vi "Read Channel Configurations.vi"(8 "error in (no error)":errorcluster, 9 "PMU Configuration":T4, 10 "PMU Index":i32, 11 "Pseudo PDC ID":i32) -> (0 "error out":errorcluster, 1 "Digital Configuration":T1, 2 "Analog Configuration":T2, 3 "Phasor Configuration":T3)   [LabVIEW 2018, in "S3DK.lvlib" / "PMU Recorder Light.lvlib" / "Statnett C37.118 DLL.lvclass"]
uses:
  Statnett C37.118 DLL.lvclass
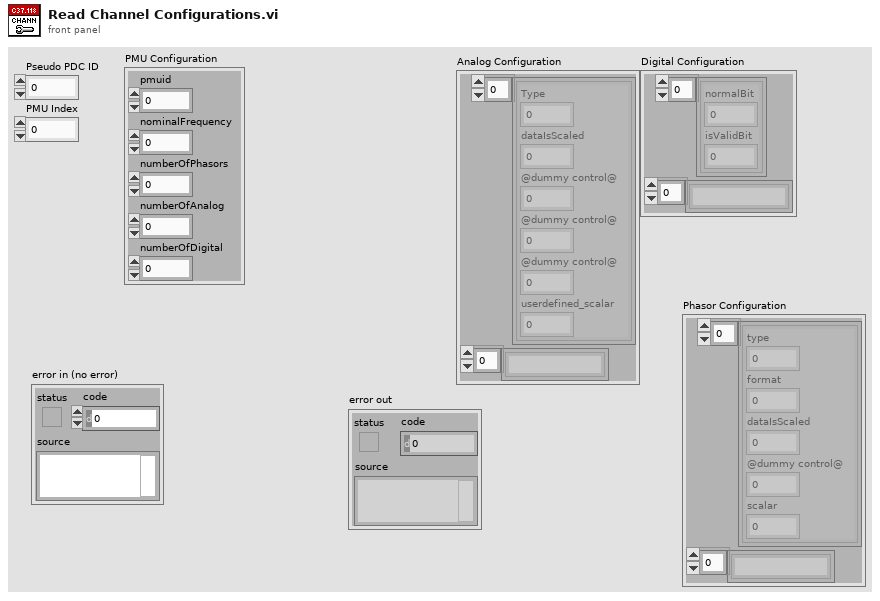
[diagram p1: front panel]
types:
  T1 = cluster{cluster{"normalBit":u8, "isValidBit":u8}[], string[]}
  T2 = cluster{cluster{"Type":i32, "dataIsScaled":u8, "@dummy control@":i8, "@dummy control@":i8, "@dummy control@":i8, "userdefined_scalar":sgl}[], string[]}
  T3 = cluster{cluster{"type":u8, "format":u8, "dataIsScaled":u8, "@dummy control@":i8, "scalar":sgl}[], string[]}
  T4 = cluster{"pmuid":i32, "nominalFrequency":sgl, "numberOfPhasors":i32, "numberOfAnalog":i32, "numberOfDigital":i32}
  T5 = cluster{"type":u8, "format":u8, "dataIsScaled":u8, "@dummy control@":i8, "scalar":sgl}
  T6 = cluster{"Type":i32, "dataIsScaled":u8, "@dummy control@":i8, "@dummy control@":i8, "@dummy control@":i8, "userdefined_scalar":sgl}
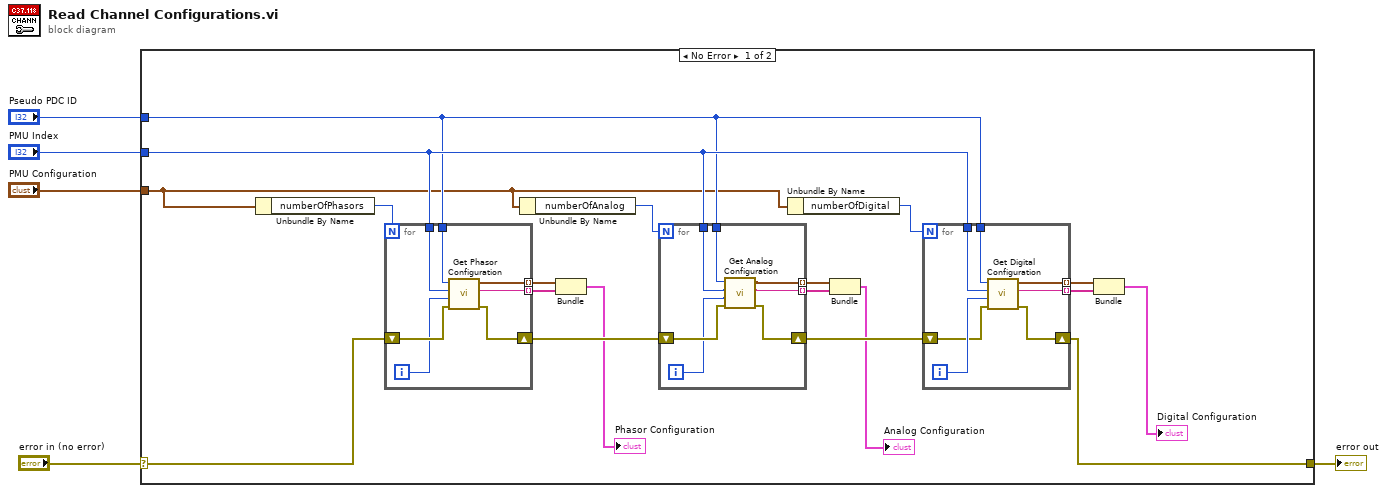
[diagram p0: block diagram]
diagram:
  n1 = case shown="No Error" "error in (no error)" {
    selector: "error in (no error)" -> [w23 w46]
    tunnel: [w12 w46] -> w4
    tunnel: "Pseudo PDC ID" -> [w15 _]
    tunnel: "PMU Index" -> [w16 _]
    tunnel: "PMU Configuration" -> [w11 _]
    frame No Error {
      n2 = Unbundle By Name(w11) -> ("numberOfPhasors"=w24:i32)
      n3 = for {
        N: w24 -> [_]
        shift-right: [w42] -> w13
        shift-left: w23 -> [w43]
        tunnel: w15 -> [w45]
        tunnel: w16 -> [w44]
        tunnel: [w41] -> w22 mode=indexing
        tunnel: [w40] -> w21 mode=indexing
        i -> [w39]
        n4 = call "Get Phasor Configuration.vi"("error in (no error)"=w43, "Phasor Index"=w39, "PMU Index"=w44, "Pseudo PDC ID"=w45) -> ("error out"=w42:errorcluster, "Phasor Name"=w40:string, "Phasor Configuration"=w41:T5)  [unwired: 5 in]
      }
      n5 = Unbundle By Name(w11) -> ("numberOfAnalog"=w10:i32)
      n6 = Bundle(w22, w21) -> (→"Phasor Configuration":T3)  [unwired: 1 in]
      n7 = for {
        N: w10 -> [_]
        shift-right: [w36] -> w14
        shift-left: w13 -> [w35]
        tunnel: w15 -> [w32]
        tunnel: w16 -> [w33]
        tunnel: [w38] -> w19 mode=indexing
        tunnel: [w37] -> w20 mode=indexing
        i -> [w34]
        n8 = call "Get Analog Configuration.vi"("error in (no error)"=w35, "Analog Index"=w34, "PMU Index"=w33, "Pseudo PDC ID"=w32) -> ("error out"=w36:errorcluster, "Analog Name"=w37:string, "Analog Configuration"=w38:T6)  [unwired: 5 in]
      }
      n9 = Unbundle By Name(w11) -> ("numberOfDigital"=w9:i32)
      n10 = Bundle(w19, w20) -> (→"Analog Configuration":T2)  [unwired: 1 in]
      n11 = for {
        N: w9 -> [_]
        shift-right: [w25] -> w12
        shift-left: w14 -> [w26]
        tunnel: w15 -> [w29]
        tunnel: w16 -> [w28]
        tunnel: [w31] -> w18 mode=indexing
        tunnel: [w30] -> w17 mode=indexing
        i -> [w27]
        n12 = call "Get Digital Configuration.vi"("error in (no error)"=w26, "Digital Index"=w27, "PMU Index"=w28, "Pseudo PDC ID"=w29) -> ("error out"=w25:errorcluster, "Digital Name"=w30:string, "Digital Configuration"=w31:cluster{"normalBit":u8, "isValidBit":u8})  [unwired: 5 in]
      }
      n13 = Bundle(w18, w17) -> (→"Digital Configuration":T1)  [unwired: 1 in]
    }
    frame Error {
    }
  }
  "error out" <- w4
